vi "Read Alicat Data.vi"(8 "error in (no error)":errorcluster, 11 "Alicat Device in":refnum<class "Alicat Device.lvclass">) -> (0 "error out":errorcluster, 2 "Alicat Data":refnum<class "Alicat Data.lvclass">, 3 "Alicat Device out":refnum<class "Alicat Device.lvclass">)   [LabVIEW 2015, in "Alicat Lib.lvlib" / "Alicat Device.lvclass"]
uses:
  Alicat Device.lvclass
  Data/Alicat Data.lvclass
  Alicat Device.lvclass/Alicat Device.ctl
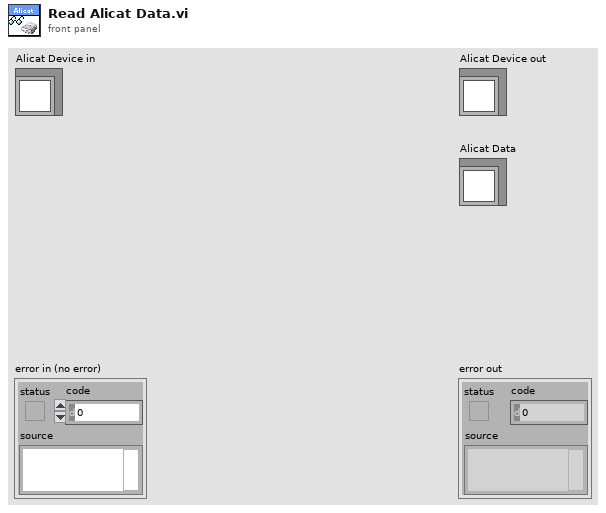
[diagram p1: front panel]
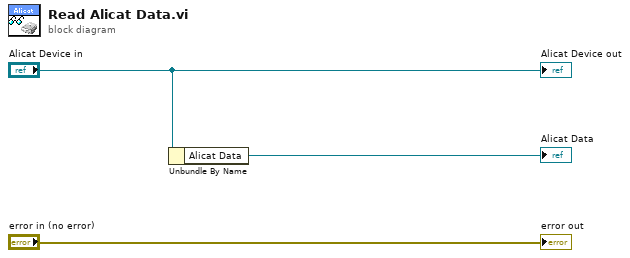
[diagram p0: block diagram]
diagram:
  n1 = Unbundle By Name("Alicat Device in") -> ("Alicat Data"=→"Alicat Data":refnum<class "Alicat Data.lvclass">)
  "error out" <- "error in (no error)"
  "Alicat Device out" <- "Alicat Device in"
